vi "Destroy Sound.vi"(8 "error in (no error)":errorcluster, 11 "Texture Name":string) -> (0 "error out":errorcluster)   [LabVIEW 2015, in "Resource Manager.lvclass"]
uses:
  Resource Manager.lvclass
  Resource Manager.lvclass/Resource Manager.ctl
  Globals.vi
  LabSDL2/Source/Libraries/LibSDL2_Mixer Wrapper/LibSDL2_Mixer.lvlib
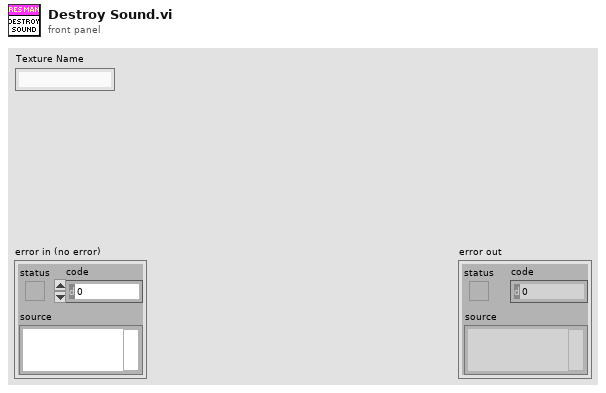
[diagram p1: front panel]
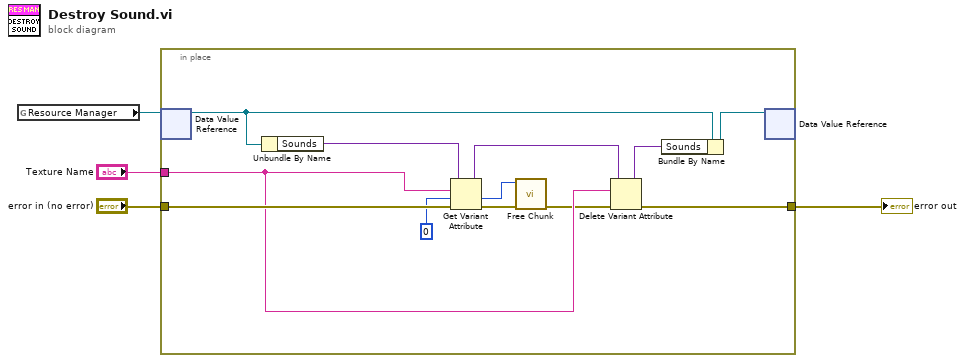
[diagram p0: block diagram]
diagram:
  n1 = global read "Globals.vi" "Resource Manager"() -> (w1:refnum<data-value>)
  n2 = in-place {
    in-place-border: "error in (no error)" -> [w15]
    in-place-border: [w13] -> w3
    in-place-border: "Texture Name" -> [w11]
    n3 = in-place-dvr #1(w1) -> (w10:refnum<class "Resource Manager.lvclass">)  [unwired: 1 out]
    n4 = Unbundle By Name(w10) -> ("Sounds"=w16:variant)
    n5 = Get Variant Attribute(Variant=w16, name=w11, default value (empty Variant)=u32 0 ("Chunk Pointer"), error in=w15) -> (duplicate Variant=w14:variant, value=w5:u32, error out=w7:errorcluster)  [unwired: 1 out]
    n6 = call "Free Chunk.vi"("error in"=w7, "Chunk Pointer"=w5) -> ("error out"=w6:errorcluster)  [unwired: 9 in]
    n7 = Delete Variant Attribute(4:w6, 6:w11, 7:w14) -> (0:w13:errorcluster, 3:w12:variant)  [unwired: 1 out]
    n8 = Bundle By Name(cluster=w10, "Sounds"=w12) -> (w9:refnum<class "Resource Manager.lvclass">)
    n9 = in-place-dvr #1(w9) -> ()  [unwired: 2 out]
  }
  "error out" <- w3
